vi "Initialise.vi"(8 "error in (no error)":errorcluster, 10 "Config":T2, 11 "Process":refnum<vi>) -> (0 "error out":errorcluster, 3 "Actor out":refnum<class "Alarms Handler Actor.lvclass">, 5 "Mailboxes":T1)   [LabVIEW 2020, in "RTAF.lvlib" / "Alarms Handler Actor.lvclass"]
uses:
  Alarms Handler Actor.lvclass
  C:/dev/PGS/2001 - TBCM/Source/RT/RTAF/Source/RTAF/Actors/Base Actor/Actor/Actor.lvclass
  Config.ctl
  API/Alarms Handler Actor API.lvclass
  C:/dev/PGS/2001 - TBCM/Source/RT/RTAF/Source/RTAF/Actors/Base Actor/API/Actor API.lvclass
  Alarms Handler Actor.lvclass/Alarms Handler Actor.ctl
  Global References.vi
  Base Actor/API/Actor API.lvclass
  Base Actor/Actor/Actor.lvclass
  RTAF.lvlib
  Base Actor/Actor/Message.ctl
  Mailboxes.ctl
  C:/dev/PGS/2001 - TBCM/Source/RT/RTAF/Source/RTAF/Actors/Alarms Handler/Actor/Alarms Handler Actor.lvclass
  C:/dev/PGS/2001 - TBCM/Source/RT/RTAF/Source/RTAF/Actors/Alarms Handler/API/Alarms Handler Actor API.lvclass
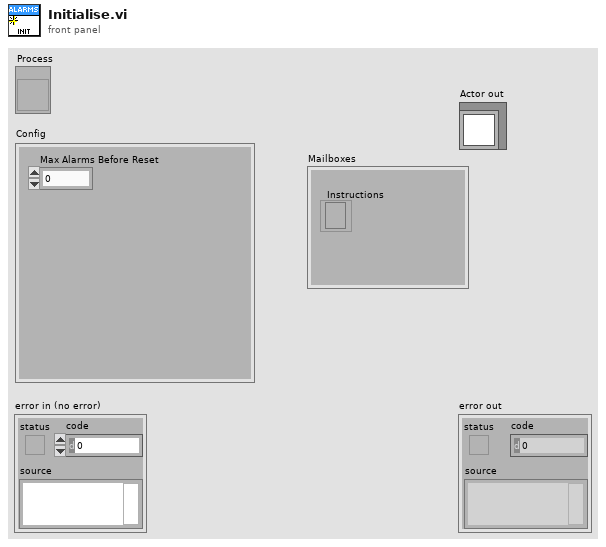
[diagram p1: front panel]
types:
  T1 = typedef "RTAF.lvlib/Alarms Handler Actor.lvclass/Mailboxes.ctl" = cluster{"Instructions":refnum<event-registration>}
  T2 = typedef "RTAF.lvlib/Alarms Handler Actor.lvclass/Config.ctl" = cluster{"Max Alarms Before Reset":i32}
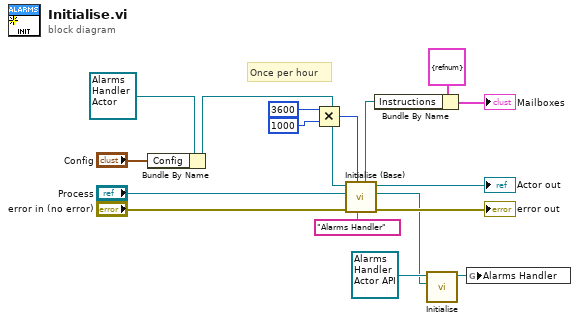
[diagram p0: block diagram]
diagram:
  # "Once per hour"
  n1 = Bundle By Name(cluster=refnum<class "Alarms Handler Actor.lvclass"> refnum ("Alarms Handler Actor.lvclass"), "Config"="Config") -> (w6:refnum<class "Alarms Handler Actor.lvclass">)
  n2 = Multiply(x=3600 ("Tick Period [100 ms]"), y=1000) -> (x*y=w11:i32)
  n3 = call "Initialise (Base).vi"("Name"="Alarms Handler", "Tick Period [100 ms]"=w11, "error in (no error)"="error in (no error)", "Process"="Process", "Actor in"=w6) -> ("error out"=→"error out":errorcluster, 2:"Instructions"=w10:refnum<user-event>, "Actor out"=→"Actor out":refnum<class "Alarms Handler Actor.lvclass">, 5:"Instructions"=w2:refnum<event-registration>)  [unwired: 3 in]
  n4 = Bundle By Name(cluster=T1 {"Instructions"=refnum} ("Mailboxes"), "Instructions"=w2) -> (→"Mailboxes":T1)
  n5 = call "Initialise.vi"("Message Channel"=w10, "Actor API in"=refnum<class "Alarms Handler Actor API.lvclass"> refnum ("Alarms Handler Actor API.lvclass")) -> ("Actor API out"=w4:refnum<class "Alarms Handler Actor API.lvclass">)  [unwired: 9 in]
  n6 = global write "Global References.vi" "Alarms Handler"(w4) -> ()
